vi "Pol2Rec9225-7_FPGA.vi"(2 "phase [pi]":fxp<+/-,36,2>, 3 "magnitude":fxp<+,36,0>) -> (0 "Im":fxp<+/-,36,0>, 1 "Re":fxp<+/-,36,0>)   [LabVIEW 2021]
uses:
  <vilib>/rvi/FXPMathLib/FxpPolarToRect/subVIs/nifxpmath_PolarToRect_SimConfig.ctl
  <vilib>/rvi/FXPMathLib/FxpPolarToRect/simVIs/DllFxpPolarToRectTemp_sub.vi
  <vilib>/rvi/FXPMathLib/FxpPolarToRect/XNode/nifxpmath_PolarToRect.xnode
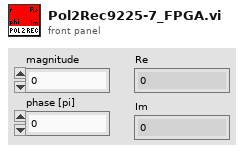
[diagram p1: front panel]
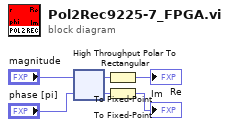
[diagram p0: block diagram]
diagram:
  n1 = xnode "High Throughput Polar To Rectangular"("magnitude"="magnitude", "phase (pi)"="phase [pi]") -> ("x"=w4:fxp<+/-,38,2>, "y"=w3:fxp<+/-,38,2>)
  n2 = To Fixed-Point(number=w4) -> (fixed-point=→"Re":fxp<+/-,36,0>)  [unwired: 1 in]
  n3 = To Fixed-Point(number=w3) -> (fixed-point=→"Im":fxp<+/-,36,0>)  [unwired: 1 in]
